vi "calibrationSpectrometer_cancelCallback_logEvent_LoopTimeOutOfRange.vi"(8 "error in (no error)":errorcluster) -> (0 "error out":errorcluster, 3 "function return":i32)   [LabVIEW 2016, in "SALLV_calibrationSpectrometer.lvlib"]
doc: "int calibrationSpectrometer_shm_cancelCallback_logevent_LoopTimeOutOfRangeLV();"
uses:
  SALLV_calibrationSpectrometer.lvlib
  SALLV_calibrationSpectrometer.so
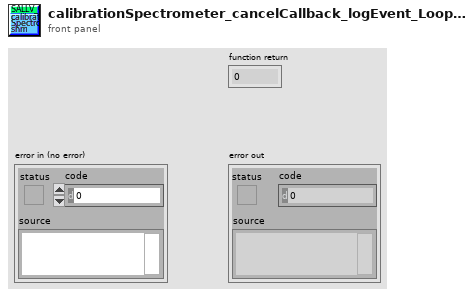
[diagram p1: front panel]
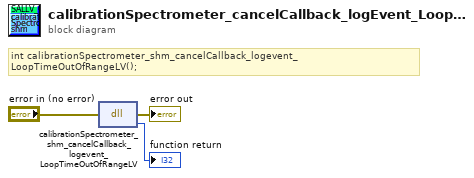
[diagram p0: block diagram]
diagram:
  # "int calibrationSpectrometer_shm_cancelCallback_logevent_LoopTimeOutOfRangeLV();"
  n1 = dll-call lib="home/harini/TCS/sallv_sedspectrometer/SALLV_calibrationSpectrometer.*" fn="calibrationSpectrometer_shm_cancelCallback_logevent_LoopTimeOutOfRangeLV"(error in="error in (no error)") -> (error out=→"error out":errorcluster, →"function return":i32)  [unwired: 2 in, 1 out]
